vi "pp2_DAQwriteAudio.vi"(5 "Daq config In":T1={"Sound AO"="Dev2/ao0", "Shock intesity AO"="Dev1/ao1", "Code_LED DO"="Dev1/port1:2", "Switch DI"="Dev1/port0/line0:1", "Webcam"="cam0", "Sound AO task"="", "Sound card task"=0, "Shock intensity AO task"="", "Code_LED DO task"="", "Switch DI task"="", "AO <=> Sound card"=FALSE, "Sound card"=0, "sample rate"=8000.0, "Variable shock"=FALSE, "Webcam on"=FALSE, "Tone gate PFI"="/Dev1/PFI1", "Waveform memo"={"t0"=timestamp(0 s since 1904-01-01), "dt"=1.0, "Y"=[]}, "First time"=FALSE} {"sample rate" min=8000.0; "Sound card task" format="%.0x"}, 7 "Waveform":waveform(dbl), 11 "error in (no error)":errorcluster) -> (6 "Daq config Out":T1={"Sound AO"="Dev2/ao0", "Shock intesity AO"="Dev1/ao1", "Code_LED DO"="Dev1/port1:2", "Switch DI"="Dev1/port0/line0:1", "Webcam"="cam0", "Sound AO task"="", "Sound card task"=0, "Shock intensity AO task"="", "Code_LED DO task"="", "Switch DI task"="", "AO <=> Sound card"=FALSE, "Sound card"=0, "sample rate"=8000.0, "Variable shock"=FALSE, "Webcam on"=FALSE, "Tone gate PFI"="/Dev1/PFI1", "Waveform memo"={"t0"=timestamp(0 s since 1904-01-01), "dt"=1.0, "Y"=[]}, "First time"=FALSE} {"sample rate" min=8000.0; "Sound card task" format="%.0x"}, 15 "error out":errorcluster)   [LabVIEW 2013]
uses:
  pp2_CTL_DaqConfig.ctl
  <vilib>/userdefined/High Color/IMAQdx.ctl
  <vilib>/sound2/lvsound2.llb/Sound Output Task ID.ctl
  <vilib>/DAQmx/create/channels.llb/DAQmx Create Channel (AO-Voltage-Basic).vi
  <vilib>/DAQmx/configure/timing.llb/DAQmx Timing (Use Waveform).vi
  <vilib>/DAQmx/write.llb/DAQmx Write (Analog Wfm 1Chan NSamp).vi
  <resource>/objmgr/daqmx.rc
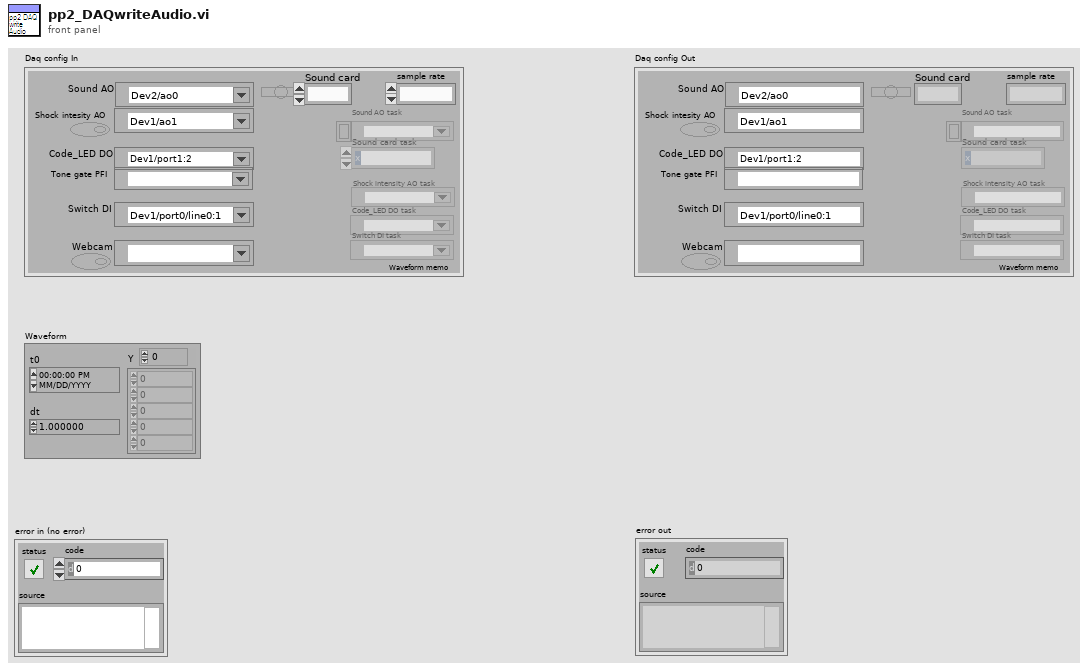
[diagram p1: front panel]
types:
  T1 = typedef "pp2_CTL_DaqConfig.ctl" = cluster{"Sound AO":tag, "Shock intesity AO":tag, "Code_LED DO":tag, "Switch DI":tag, "Webcam":T2, "Sound AO task":refnum<k21>, "Sound card task":T3, "Shock intensity AO task":refnum<k21>, "Code_LED DO task":refnum<k21>, "Switch DI task":refnum<k21>, "AO <=> Sound card":bool, "Sound card":u32, "sample rate":dbl, "Variable shock":bool, "Webcam on":bool, "Tone gate PFI":tag, "Waveform memo":waveform(dbl), "First time":bool}
  T2 = typedef "IMAQdx.ctl" = refnum<k21>
  T3 = typedef "Sound Output Task ID.ctl" = u32
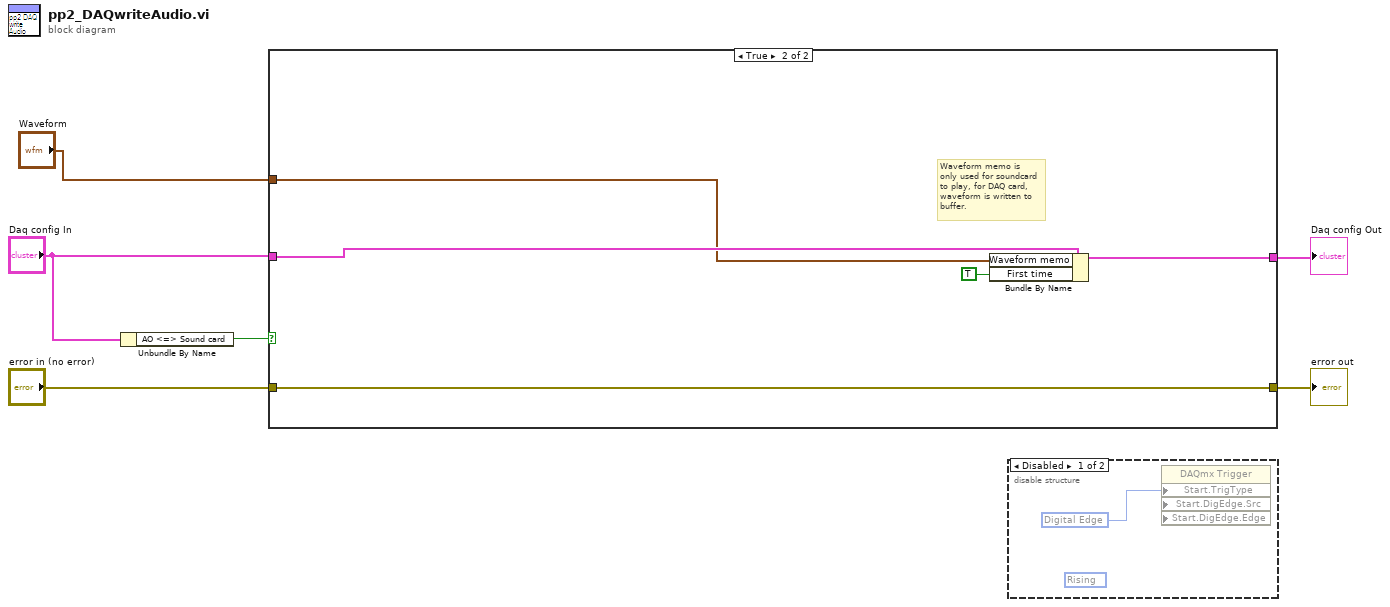
[diagram p0: block diagram]
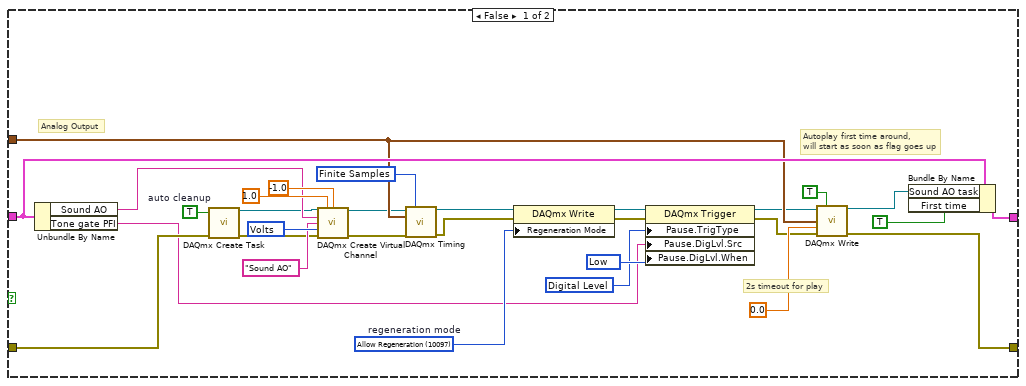
[diagram p3: hidden frame]
diagram:
  n1 = Unbundle By Name("Daq config In") -> ("AO <=> Sound card"=w6:bool)
  n2 = case shown="True" w6 {
    tunnel: "Daq config In" -> [w35 w40]
    tunnel: [w34 w41] -> w3
    tunnel: "error in (no error)" -> [w17 w38]
    tunnel: [w32 w38] -> w2
    tunnel: "Waveform" -> [w30 w39]
    frame False {
      w10 = 10214 items=["High"=10192, "Low"=10214] ("Pause.DigLvl.When")
      w9 = 10152 items=["Analog Level"=10101, "Analog Window"=10103, "Digital Level"=10152, "Digital Pattern"=10398, "None"=10230] ("Pause.TrigType")
      w19 = TRUE  # auto cleanup
      w20 = 10097 items=["Allow Regeneration"=10097, "Do Not Allow Regeneration"=10158]  # regeneration mode
      w29 = 10348 items=["Volts"=10348, "From Custom Scale"=10065] ("units")
      w31 = 10178 items=["Finite Samples"=10178, "Continuous Samples"=10123, "Hardware Timed Single Point"=12522] ("sample mode")
      # "2s timeout for play"
      # "Autoplay first time around,\nwill start as soon as flag goes up"
      # "Analog Output"
      n3 = Unbundle By Name(w35) -> ("Sound AO"=w23:tag, "Tone gate PFI"=w8:tag)
      n4 = call <vilib>:"DAQmx Create Task.vi"("auto cleanup"=w19, "error in"=w17) -> ("task out"=w18:refnum<k21>, "error out"=w16:errorcluster)  [unwired: 12 in]
      n5 = call-poly <vilib>:"DAQmx Create Virtual Channel.vi"("task in"=w18, "maximum value"=1.0, "minimum value"=-1.0, "physical channels"=w23, "name to assign"="Sound AO", "units"=w29, "error in"=w16) -> ("task out"=w25:refnum<k21>, "error out"=w24:errorcluster)  [unwired: 7 in]
      n6 = call-poly <vilib>:"DAQmx Timing.vi"("task/channels in"=w25, "sample mode"=w31, "waveform"=w30, "error in"=w24) -> ("task out"=w22:refnum<k21>, "error out"=w21:errorcluster)  [unwired: 10 in]
      n7 = property class="DAQmx Write"(reference=w22, error in=w21, "Regeneration Mode"=w20) -> (reference out=w14:refnum<k21>, error out=w13:errorcluster)
      n8 = property class="DAQmx Trigger"(reference=w14, error in=w13, "Pause.TrigType"=w9, "Pause.DigLvl.Src"=w8, "Pause.DigLvl.When"=w10) -> (reference out=w12:refnum<k21>, error out=w11:errorcluster)
      n9 = call-poly <vilib>:"DAQmx Write.vi"("task/channels in"=w12, "auto start"=TRUE, "data"=w30, "timeout"=0.0, "error in"=w11) -> ("task out"=w33:refnum<k21>, "error out"=w32:errorcluster)  [unwired: 8 in, 1 out]
      n10 = Bundle By Name(cluster=w35, "Sound AO task"=w33, "First time"=TRUE) -> (w34:T1)
    }
    frame True {
      # "Waveform memo is\nonly used for soundcard\nto play, for DAQ card,\nwaveform is written to\nbuffer."
      n11 = Bundle By Name(cluster=w40, "Waveform memo"=w39, "First time"=TRUE) -> (w41:T1)
    }
  }
  "Daq config Out" <- w3
  "error out" <- w2
  n12 = disable-structure shown="Disabled" {
    frame Disabled {
      w42 = 10280 items=["Rising"=10280, "Falling"=10171] ("Start.DigEdge.Edge")
      w43 = 10150 items=["Analog Edge"=10099, "Digital Edge"=10150, "Digital Pattern"=10398, "Analog Window"=10103, "None"=10230] ("Start.TrigType")
      n13 = property class="DAQmx Trigger" props=["Start.TrigType", "Start.DigEdge.Src", "Start.DigEdge.Edge"]("Start.TrigType"=w43) -> ()  [unwired: 4 in, 2 out]
    }
    frame Enabled {
    }
  }
